vi "Read FW INI.vi"(8 "Error In":errorcluster, 11 "Firmware INI Path":path) -> (0 "Error Out":errorcluster, 2 "Firmware Config":T1, 3 "Duplicate Firmware INI Path":path)   [LabVIEW 2020, in "LMH-LINX.lvlib"]
uses:
  LMH-LINX.lvlib
  Type Defs/Device Firmware.ctl
  <vilib>/Utility/config.llb/Read Key (String).vi
  <vilib>/Utility/config.llb/Read Key (I32).vi
  <vilib>/Utility/config.llb/Read Key (Path).vi
  <vilib>/Utility/config.llb/NI_LVConfig.lvlib
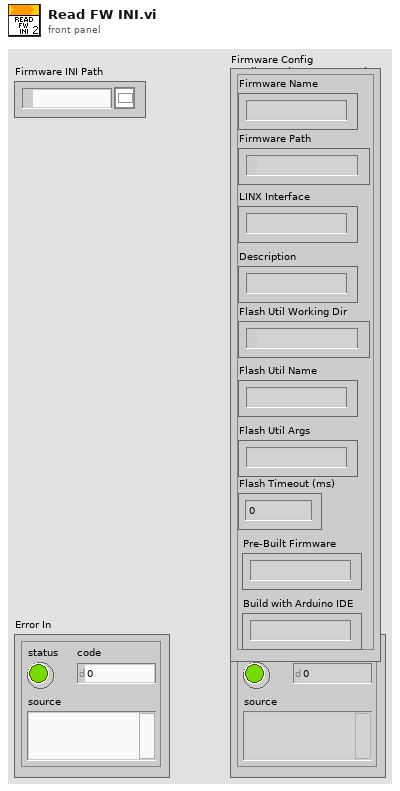
[diagram p1: front panel]
types:
  T1 = typedef "LMH-LINX.lvlib/Device Firmware.ctl" = cluster{"Firmware Name":string, "Firmware Path":path, "Description":string, "LINX Interface":string, "Flash Util Working Dir":path, "Flash Util Name":string, "Flash Util Args":string, "Flash Timeout (ms)":i32, "Pre-Built Firmware":string, "Build with Arduino IDE":string}
  T2 = typedef "NI_LVConfig.lvlib/Config Data RefNum.ctl" = refnum<k1>
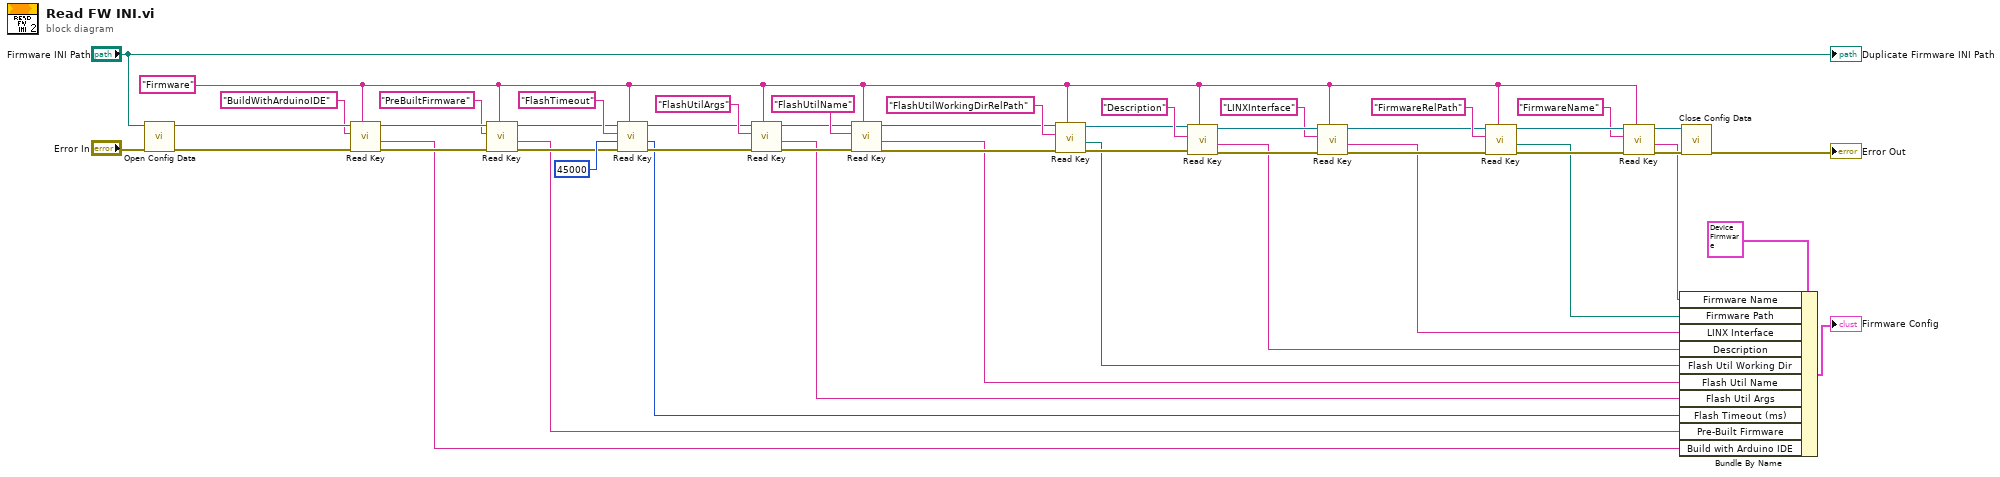
[diagram p0: block diagram]
diagram:
  w5 = "Firmware" ("key")
  n1 = call <vilib>:"Open Config Data.vi"("error in (no error)"="Error In", "configuration file path"="Firmware INI Path") -> ("error out"=w10:errorcluster, "refnum"=w11:T2)  [unwired: 7 in, 1 out]
  n2 = call-poly <vilib>:"Read Key.vi"("section"=w5, "error in (no error)"=w10, "key"="BuildWithArduinoIDE", "refnum"=w11) -> ("error out"=w8:errorcluster, "value"=w1:string, "refnum out"=w9:T2)  [unwired: 4 in, 1 out]
  n3 = call-poly <vilib>:"Read Key.vi"("section"=w5, "error in (no error)"=w8, "key"="PreBuiltFirmware", "refnum"=w9) -> ("error out"=w7:errorcluster, "value"=w2:string, "refnum out"=w6:T2)  [unwired: 4 in, 1 out]
  n4 = call-poly <vilib>:"Read Key.vi"("section"=w5, "error in (no error)"=w7, "default value"=45000, "key"="FlashTimeout", "refnum"=w6) -> ("error out"=w15:errorcluster, "value"=w12:i32, "refnum out"=w14:T2)  [unwired: 3 in, 1 out]
  n5 = call-poly <vilib>:"Read Key.vi"("section"=w5, "error in (no error)"=w15, "key"="FlashUtilArgs", "refnum"=w14) -> ("error out"=w23:errorcluster, "value"=w17:string, "refnum out"=w22:T2)  [unwired: 4 in, 1 out]
  n6 = call-poly <vilib>:"Read Key.vi"("section"=w5, "error in (no error)"=w23, "key"="FlashUtilName", "refnum"=w22) -> ("error out"=w24:errorcluster, "value"=w18:string, "refnum out"=w21:T2)  [unwired: 4 in, 1 out]
  n7 = call-poly <vilib>:"Read Key.vi"("section"=w5, "error in (no error)"=w24, "key"="FlashUtilWorkingDirRelPath", "refnum"=w21) -> ("error out"=w25:errorcluster, "value"=w19:path, "refnum out"=w20:T2)  [unwired: 4 in, 1 out]
  n8 = call-poly <vilib>:"Read Key.vi"("section"=w5, "error in (no error)"=w25, "key"="Description", "refnum"=w20) -> ("error out"=w40:errorcluster, "value"=w29:string, "refnum out"=w41:T2)  [unwired: 4 in, 1 out]
  n9 = call-poly <vilib>:"Read Key.vi"("section"=w5, "error in (no error)"=w40, "key"="LINXInterface", "refnum"=w41) -> ("error out"=w31:errorcluster, "value"=w30:string, "refnum out"=w32:T2)  [unwired: 4 in, 1 out]
  n10 = call-poly <vilib>:"Read Key.vi"("section"=w5, "error in (no error)"=w31, "key"="FirmwareRelPath", "refnum"=w32) -> ("error out"=w39:errorcluster, "value"=w34:path, "refnum out"=w42:T2)  [unwired: 4 in, 1 out]
  n11 = call-poly <vilib>:"Read Key.vi"("section"=w5, "error in (no error)"=w39, "key"="FirmwareName", "refnum"=w42) -> ("error out"=w44:errorcluster, "value"=w37:string, "refnum out"=w43:T2)  [unwired: 4 in, 1 out]
  n12 = Bundle By Name(cluster=T1 {"Firmware Name"="", "Firmware Path"=path "", "Description"="", "LINX Interface"="", "Flash Util Working Dir"=path "", "Flash Util Name"="", "Flash Util Args"="", "Flash Timeout (ms)"=0, "Pre-Built Firmware"="", "Build with Arduino IDE"=""} ("Device Firmware"), "Firmware Name"=w37, "Firmware Path"=w34, "LINX Interface"=w30, "Description"=w29, "Flash Util Working Dir"=w19, "Flash Util Name"=w18, "Flash Util Args"=w17, "Flash Timeout (ms)"=w12, "Pre-Built Firmware"=w2, "Build with Arduino IDE"=w1) -> (→"Firmware Config":T1)
  n13 = call <vilib>:"Close Config Data.vi"("error in (no error)"=w44, "refnum"=w43) -> ("error out"=→"Error Out":errorcluster)  [unwired: 8 in, 1 out]
  "Duplicate Firmware INI Path" <- "Firmware INI Path"
